vi "Go to LeafNode.vi"(8 "error in":errorcluster caption="错误输入（无错误）", 10 "LeafNumber":string, 11 "PanelLinkNode 输入":refnum<class "PanelLinkNode.lvclass"> caption="DNL_LabVIEW Object in") -> (0 "error out":errorcluster caption="错误输出", 1 "is rootnode?":bool, 2 "Node*":refnum<data-value>, 3 "PanelLinkNode 输出":refnum<class "PanelLinkNode.lvclass"> caption="DNL_LabVIEW Object out")   [LabVIEW 2016, in "PanelLinkNode.lvclass"]
uses:
  PanelLinkNode.lvclass
  PanelObject/PanelObject.lvclass
  PanelLinkNode.lvclass/PanelLinkNode.ctl
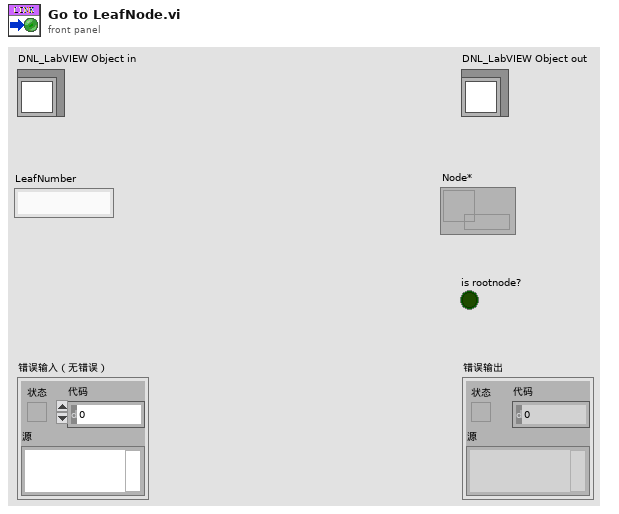
[diagram p1: front panel]
types:
  T1 = cluster{"NodePath/Number":string, "Node*":refnum<data-value>}
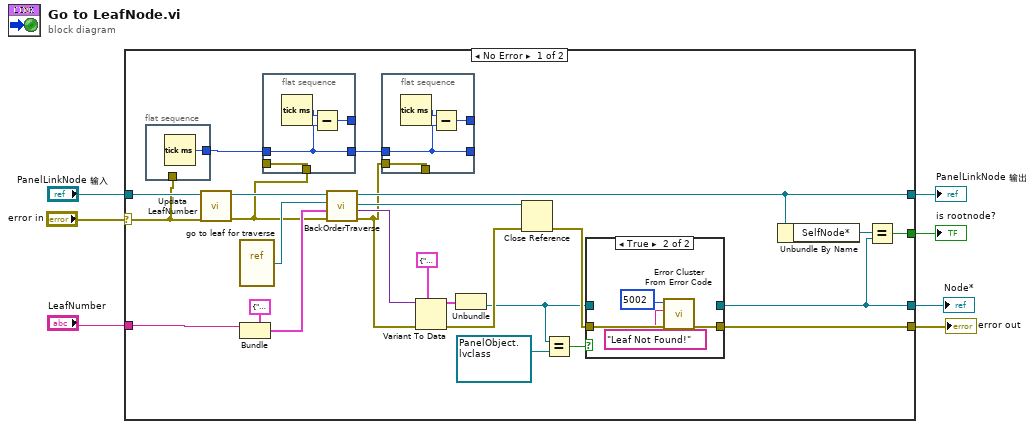
[diagram p0: block diagram]
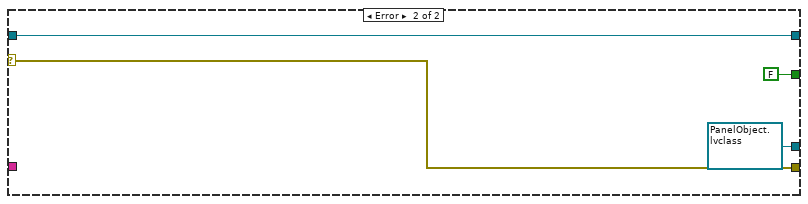
[diagram p3: hidden frame]
diagram:
  n1 = case shown="No Error" "error in" {
    selector: "error in" -> [w12 w51]
    tunnel: [w31 w51] -> w6
    tunnel: [w19 w50] -> w4
    tunnel: "PanelLinkNode 输入" -> [w14 w50]
    tunnel: [w15 refnum<data-value> refnum ("Node*")] -> w1
    tunnel: "LeafNumber" -> [w28 _]
    tunnel: [w16 FALSE] -> w2
    frame No Error {
      n2 = flat-sequence {
        tunnel: [w41] -> w11
        tunnel: w12 -> [_]
        frame #0 {
          n3 = Tick Count (ms)() -> (millisecond timer value=w41:u32)
        }
      }
      n4 = call-dynamic "Updata LeafNumber.vi"("error in (no error)"=w12, "PanelLinkNode 输入"=w14) -> ("error out"=w10:errorcluster, "PanelLinkNode 输出"=w13:refnum<class "PanelLinkNode.lvclass">)  [unwired: 7 in, 1 out]
      n5 = vi-ref "go to leaf for traverse.vi"() -> (w23:refnum<vi>)
      n6 = Bundle(cluster=T1 {"NodePath/Number"="", "Node*"=refnum} ("Data out"), "NodePath/Number"=w28) -> (w27:T1)  [unwired: 1 in]
      n7 = flat-sequence {
        tunnel: [w39] -> w8
        tunnel: w11 -> [w39]
        tunnel: [w38] -> _
        tunnel: [w37] -> _
        tunnel: w10 -> [w37]
        frame #0 {
          n8 = Tick Count (ms)() -> (millisecond timer value=w40:u32)
          n9 = Subtract(x=w40, y=w39) -> (x-y=w38:u32)
        }
      }
      n10 = call-dynamic "BackOrderTraverse.vi"("error in"=w10, "Data in"=w27, "vi reference"=w23, "PanelLinkNode 输入"=w13) -> ("error out"=w9:errorcluster, "Data out"=w32:variant, "vi reference out"=w20:refnum<vi>, "PanelLinkNode 输出"=w19:refnum<class "PanelLinkNode.lvclass">)  [unwired: 3 in, 1 out]
      n11 = flat-sequence {
        tunnel: [w35] -> _
        tunnel: w8 -> [w35]
        tunnel: [w34] -> _
        tunnel: w9 -> [w33]
        tunnel: [w33] -> _
        frame #0 {
          n12 = Tick Count (ms)() -> (millisecond timer value=w36:u32)
          n13 = Subtract(x=w36, y=w35) -> (x-y=w34:u32)
        }
      }
      n14 = Variant To Data(error in=w9, type=T1 {"NodePath/Number"="", "Node*"=refnum} ("Data out"), Variant=w32) -> (data=w26:T1, error out=w22:errorcluster)
      n15 = Unbundle(w26) -> ("Node*"=w17:refnum<data-value>)  [unwired: 1 out]
      n16 = Close Reference(reference=w20, error in (no error)=w22) -> (error out=w21:errorcluster)
      n17 = Equal?(x=w17, y=refnum<data-value> refnum) -> (x = y?=w24:bool)
      n18 = case shown="True" w24 {
        tunnel: [w43 _] -> w15
        tunnel: w21 -> [w42 w46]
        tunnel: [w42 w47] -> w31
        tunnel: w17 -> [w43 _]
        frame False {
        }
        frame True {
          n19 = call <vilib>:"Error Cluster From Error Code.vi"("error in (no error)"=w46, "error message (\"\")"="Leaf Not Found!" ("error message (\"\")"), "error code (0)"=5002) -> ("error out"=w47:errorcluster)  [unwired: 6 in]
        }
      }
      n20 = Unbundle By Name(w19) -> ("SelfNode*"=w18:refnum<data-value>)
      n21 = Equal?(x=w18, y=w15) -> (x = y?=w16:bool)
    }
    frame Error {
    }
  }
  "error out" <- w6
  "PanelLinkNode 输出" <- w4
  "is rootnode?" <- w2
  "Node*" <- w1
